vi "X轴连续扫描（1.0）.vi"(0 "VISA I":refnum<visa-resource-name>, 2 "X0":dbl, 3 "X":dbl, 4 "精度":dbl=0.001, 5 "细分设置":dbl=8.0, 6 "等待时间(ms)":u32=40, 7 "pulDDR2Length":u32, 8 "电机急停":bool, 9 "hDevice":i32, 11 "M-length":dbl, 13 "N-length":dbl) -> (14 "VISA O":refnum<visa-resource-name>, 15 "hDevice out":i32, 16 "X":dbl, 17 "强度图行":dbl[](array[numeric]), 18 "时域谱页":dbl[][](array[numeric]), 19 "幅频谱页":dbl[][](array[numeric]))   [LabVIEW 2016]
panel:
  out "大小":i32[](array[numeric])
  out "幅频谱":dbl[](graph)
  out "时域谱":dbl[](graph)
  # "X："
  # "时域谱"
  # "频域谱"
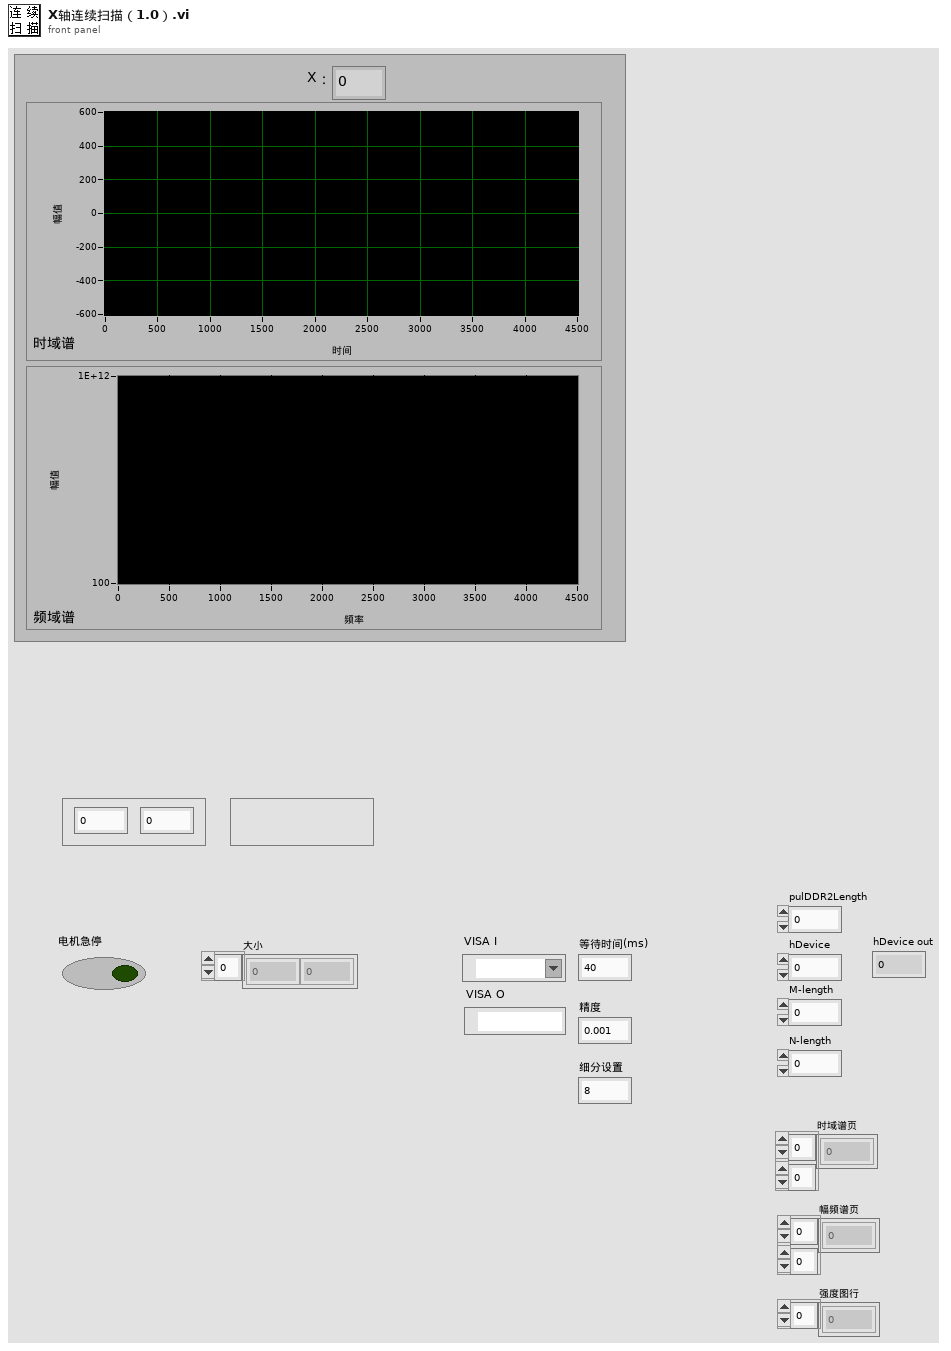
[diagram p1: front panel]
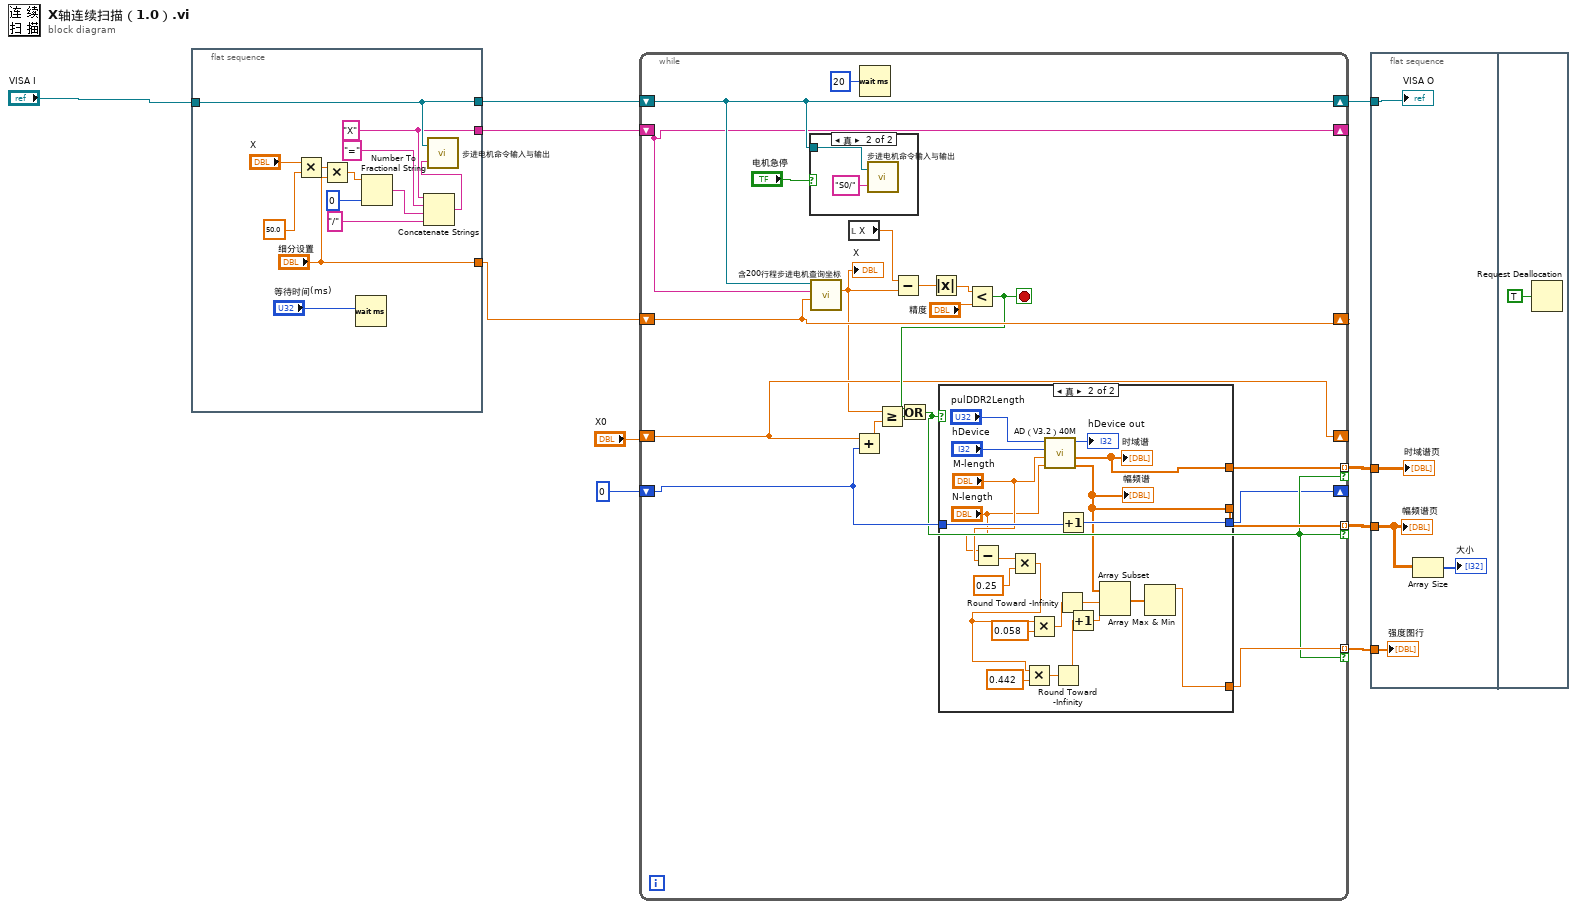
[diagram p0: block diagram]
diagram:
  n1 = flat-sequence {
    tunnel: "VISA I" -> [w15]
    tunnel: [w15] -> w9
    tunnel: ["细分设置"] -> w7
    tunnel: [w12] -> w8
    frame #0 {
      w12 = "X"
      n2 = Multiply(x="X", y=50.0 ("x")) -> (x*y=w18:dbl)
      n3 = Multiply(x=w18, y="细分设置") -> (x*y=w23:dbl)
      n4 = Wait (ms)(milliseconds to wait="等待时间(ms)") -> ()  [unwired: 1 out]
      n5 = Number To Fractional String(number=w23, precision (6)=i16 0 ("精度(6)")) -> (F-format string=w21:string)  [unwired: 2 out]
      n6 = Concatenate Strings(w12, "=" ("字符串"), w21, "/" ("字符串")) -> (w17:string)
      n7 = call "步进电机命令输入与输出.vi"("输入字符串"=w17, "串口通信端口"=w15) -> ()  [unwired: 1 out]
    }
  }
  n8 = while {
    shift-right: [w41] -> w2
    shift-left: w9 -> [w41]
    shift-right: [w25] -> _
    shift-left: "X0" -> [w25]
    shift-right: [w35] -> _
    shift-left: w7 -> [w35]
    shift-right: [w27] -> _
    shift-left: w8 -> [w27]
    tunnel: [w34] -> w3 mode=indexing if=w29
    shift-right: [w26] -> _
    shift-left: 0 -> [w33]
    tunnel: [w32] -> w5 mode=indexing if=w29
    tunnel: [w31] -> w4 mode=indexing if=w29
    stop <- w28 stop-if-true
    n9 = case shown="真" "电机急停" {
      tunnel: w41 -> [_ w66]
      frame False {
      }
      frame True {
        n10 = call "步进电机命令输入与输出.vi"("输入字符串"="S0/", "串口通信端口"=w66) -> ()  [unwired: 1 out]
      }
    }
    n11 = call "含200行程步进电机查询坐标.vi"("细分设置"=w35, "查询坐标轴"=w27, "串口通信端口"=w41) -> ("坐标(mm)"=w24:dbl)  [unwired: 8 in]
    "X" <- w24
    n12 = local read "X"() -> (w37:dbl)
    n13 = Add(x=w25, y=w33) -> (x+y=w36:dbl)
    n14 = Wait (ms)(milliseconds to wait=u32 20 ("等待时间（毫秒）")) -> ()  [unwired: 1 out]
    n15 = Greater Or Equal?(x=w24, y=w36) -> (x >= y?=w30:bool)
    n16 = Subtract(x=w37, y=w24) -> (x-y=w43:dbl)
    n17 = Absolute Value(x=w43) -> (abs(x)=w42:dbl)
    n18 = Less?(x=w42, y="精度") -> (x < y?=w28:bool)
    n19 = Or(x=w28, y=w30) -> (x .or. y?=w29:bool)
    n20 = case shown="真" w29 {
      tunnel: [_ w46] -> w34
      tunnel: w33 -> [w44 w62]
      tunnel: [w44 w61] -> w26
      tunnel: [_ w60] -> w32
      tunnel: [_ w45] -> w31
      frame False {
      }
      frame True {
        n21 = Subtract(x="N-length", y="M-length") -> (x-y=w58:dbl)
        n22 = Multiply(x=w58, y=0.25) -> (x*y=w48:dbl)
        n23 = Multiply(x=w48, y=0.442) -> (x*y=w51:dbl)
        n24 = Multiply(x=w48, y=0.058) -> (x*y=w53:dbl)
        n25 = call "AD（V3.2）40M.vi"("N-length"="N-length", "M-length"="M-length", "hDevice"="hDevice", "pulDDR2Length"="pulDDR2Length") -> ("幅频谱"=w46:dbl[], "时域谱"=w60:dbl[], "hDevice out"=→"hDevice out":i32)  [unwired: 5 in]
        "时域谱" <- w60
        "幅频谱" <- w46
        n26 = Round Toward -Infinity(1:w51) -> (0:w49:dbl)
        n27 = Round Toward -Infinity(1:w53) -> (0:w52:dbl)
        n28 = Increment(x=w62) -> (x+1=w61:i32)
        n29 = Increment(x=w49) -> (x+1=w55:dbl)
        n30 = Array Subset(array=w46, index=w52, length=w55) -> (w47:dbl[])
        n31 = Array Max & Min(array=w47) -> (max value=w45:dbl)  [unwired: 3 out]
      }
    }
  }
  n32 = flat-sequence {
    tunnel: w5 -> [w72]
    tunnel: w4 -> [w71]
    tunnel: w3 -> [w70]
    tunnel: w2 -> [w68]
    frame #0 {
      n33 = Array Size(array=w70) -> (size(s)=→"大小":i32[])
      "VISA O" <- w68
      "幅频谱页" <- w70
      "时域谱页" <- w72
      "强度图行" <- w71
    }
    frame #1 {
      n34 = Request Deallocation(TRUE ("标志")) -> ()
    }
  }
